vi "Update IODevInfo.vi"(8 "error in (no error)":errorcluster, 10 "IODevInfo":refnum<class "IODevInfo.lvclass">, 11 "Sequencer in":refnum<class "Sequencer.lvclass">) -> (0 "error out":errorcluster, 3 "Sequencer out":refnum<class "Sequencer.lvclass">)   [LabVIEW 2015, in "Sequencer.lvlib" / "Sequencer.lvclass"]
uses:
  Sequencer.lvclass
  IO Device/IODevInfo.lvclass
  IO Device/IODevConfig.lvclass
  SequencerInfo.lvclass
  SequencerConfig.lvclass
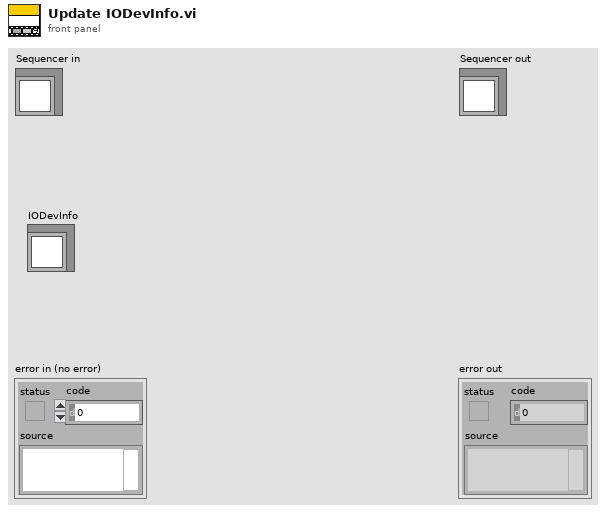
[diagram p1: front panel]
types:
  T1 = typedef "Sequencer.lvlib/Sequencer.lvclass/Daq Channel Info.ctl" = cluster{"DevNames":tag[], "AO.PhysicalChans":tag[][], "DO.Lines":tag[][], "AI.PhysicalChans":tag[][]}
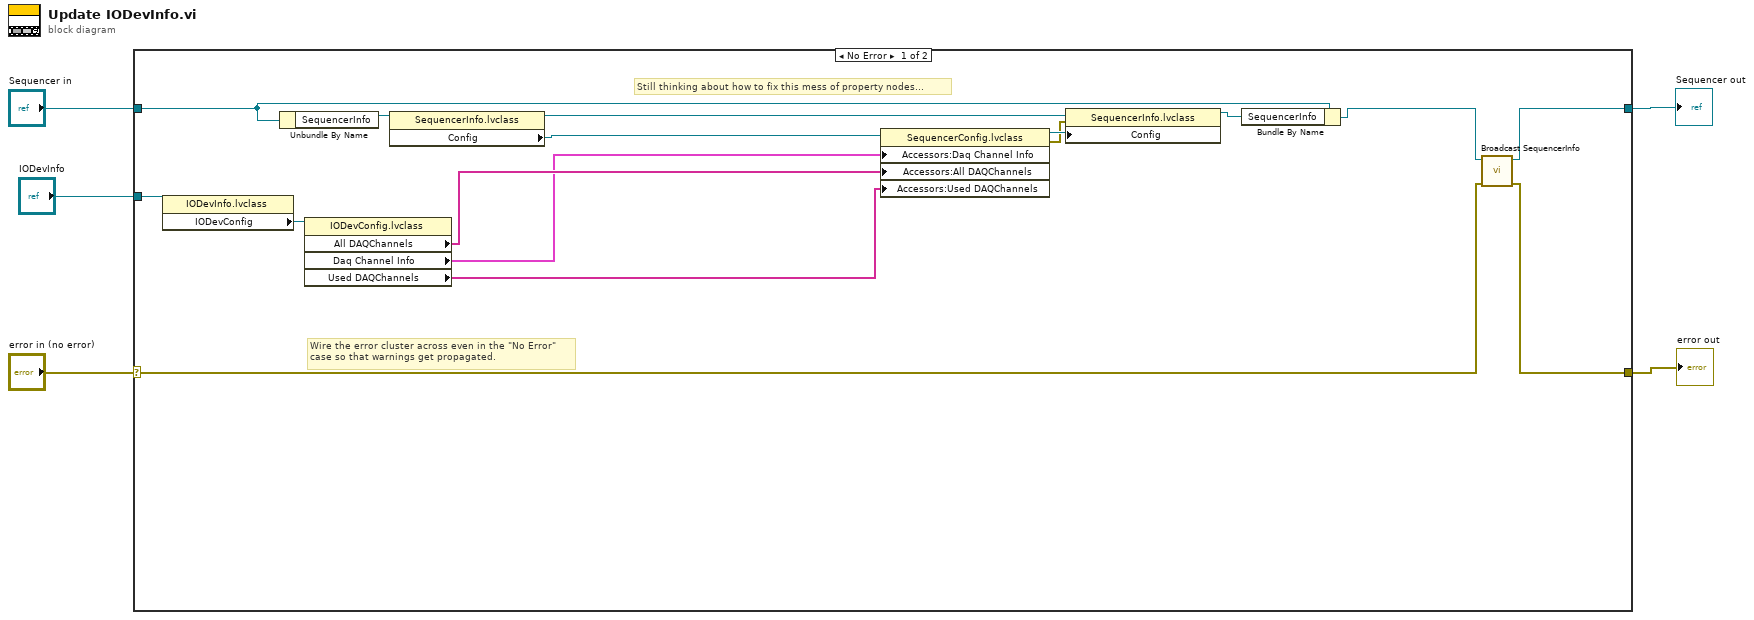
[diagram p0: block diagram]
diagram:
  n1 = case shown="No Error" "error in (no error)" {
    selector: "error in (no error)" -> [w7 w23]
    tunnel: [w6 w23] -> w4
    tunnel: [w8 w22] -> w2
    tunnel: "Sequencer in" -> [w14 w22]
    tunnel: "IODevInfo" -> [w21 _]
    frame No Error {
      # "Still thinking about how to fix this mess of property nodes..."
      # "Wire the error cluster across even in the \"No Error\"\ncase so that warnings get propagated."
      n2 = property class="IODevInfo.lvclass"(reference=w21) -> ("IODevConfig"=w20:refnum<class "IODevConfig.lvclass">)  [unwired: 1 in, 2 out]
      n3 = Unbundle By Name(w14) -> ("SequencerInfo"=w19:refnum<class "SequencerInfo.lvclass">)
      n4 = property class="IODevConfig.lvclass"(reference=w20) -> ("All DAQChannels"=w12:tag[], "Daq Channel Info"=w11:T1, "Used DAQChannels"=w10:tag[])  [unwired: 1 in, 2 out]
      n5 = property class="SequencerInfo.lvclass"(reference=w19) -> (reference out=w16:refnum<class "SequencerInfo.lvclass">, "Config"=w13:refnum<class "SequencerConfig.lvclass">)  [unwired: 1 in, 1 out]
      n6 = property class="SequencerConfig.lvclass"(reference=w13, "Accessors:Daq Channel Info"=w11, "Accessors:All DAQChannels"=w12, "Accessors:Used DAQChannels"=w10) -> (reference out=w18:refnum<class "SequencerConfig.lvclass">, error out=w15:errorcluster)  [unwired: 1 in]
      n7 = property class="SequencerInfo.lvclass"(reference=w16, error in=w15, "Config"=w18) -> (reference out=w17:refnum<class "SequencerInfo.lvclass">)  [unwired: 1 out]
      n8 = Bundle By Name(cluster=w14, "SequencerInfo"=w17) -> (w9:refnum<class "Sequencer.lvclass">)
      n9 = call "Broadcast SequencerInfo.vi"("error in (no error)"=w7, "Sequencer in"=w9) -> ("error out"=w6:errorcluster, "Sequencer out"=w8:refnum<class "Sequencer.lvclass">)  [unwired: 8 in]
    }
    frame Error {
    }
  }
  "error out" <- w4
  "Sequencer out" <- w2
